vi "Export - Buffered Rx Packet.vi"(8 "error in (no error)":errorcluster, 11 "Device Item Ref in":T10 format="%.0x") -> (0 "error out":errorcluster, 3 "Rx Packet":T1 {"targetPriority" min=-2 max=16 step=1; "targetProcessor" min=-2 max=16 step=1; "Endianness" items=["big-endian"=0, "little-endian"=2]})   [LabVIEW 2019, in "UDP-Custom-Device System Explorer.lvlib"]
uses:
  UDP-Custom-Device System Explorer.lvlib
  <vilib>/NI VeriStand/Custom Device API/Custom Device Item Ref.ctl
  Types/XML - New/ImpExp - Rx Packet Data.ctl
  <vilib>/NI VeriStand/Custom Device API/Custom Device Item Info.ctl
  Shared/Types/Shared - Channel Data Type.ctl
  Shared/Types/Shared - Buffered.PacketInfo.ctl
  Shared/Types/Shared - Pointer Encoding.ctl
  Shared/Types/Shared - Receive Buffer Options.ctl
  Shared/Types/Shared - Transmit Buffer Options.ctl
  Shared/Types/Shared - New Data Options.ctl
  Shared/Types/Shared - Thread Management.ctl
  Shared/UDP-Custom-Device Shared.lvlib
  <vilib>/NI VeriStand/Custom Device API/Custom Device API.lvlib
  Property Accessors/Shared Packet Accessors.lvlib
  Property Accessors/Rx Packet Accessors.lvlib
  Property Accessors/Buffered Data Packet.lvlib
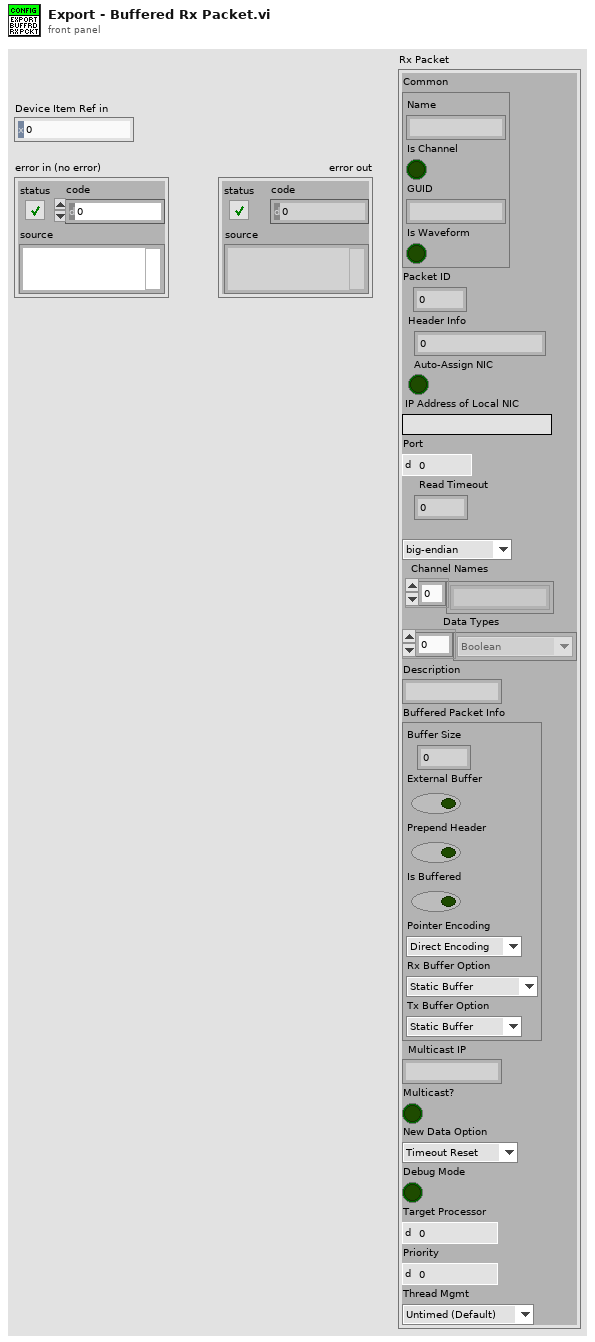
[diagram p1: front panel]
types:
  T1 = typedef "UDP-Custom-Device System Explorer.lvlib/ImpExp - Rx Packet Data.ctl" = cluster{"Common":T2, "Packet ID":i32, "Header Info":u32, "Auto-Assign NIC":bool, "IP Address of Local NIC":string, "Port":u16, "Read Timeout":i32, "Endianness":u16, "Channel Names":string[], "Data Types":T3[], "Description":string, "Buffered Packet Info":T4, "Multicast IP":string, "Multicast?":bool, "New Data Option":T8, "Debug Mode":bool, "targetProcessor":i8, "targetPriority":i16, "Thread Mgmt":T9}
  T2 = typedef "Custom Device API.lvlib/Custom Device Item Info.ctl" = cluster{"Name":string, "Is Channel":bool, "GUID":string, "Is Waveform":bool}
  T3 = typedef "UDP-Custom-Device Shared.lvlib/Shared - Channel Data Type.ctl" = enum16{"Boolean", "Single", "Double", "I8", "I16", "I32", "I64", "U8", "U16", "U32", "U64"}
  T4 = typedef "UDP-Custom-Device Shared.lvlib/Shared - Buffered.PacketInfo.ctl" = cluster{"Buffer Size":i32, "External Buffer":bool, "Prepend Header":bool, "Is Buffered":bool, "Pointer Encoding":T5, "Rx Buffer Option":T6, "Tx Buffer Option":T7}
  T5 = typedef "UDP-Custom-Device Shared.lvlib/Shared - Pointer Encoding.ctl" = enum16{"Direct Encoding", "Conversion Encoding"}
  T6 = typedef "UDP-Custom-Device Shared.lvlib/Shared - Receive Buffer Options.ctl" = enum16{"Static Buffer", "Circular Buffer", "Circular Buffer + Size", "Internal Cache", "Internal Cache + Size", "Ping Pong", "Ping Pong + Size"}
  T7 = typedef "UDP-Custom-Device Shared.lvlib/Shared - Transmit Buffer Options.ctl" = enum16{"Static Buffer", "FIFO Buffer", "FIFO Buffer + Port"}
  T8 = typedef "UDP-Custom-Device Shared.lvlib/Shared - New Data Options.ctl" = enum16{"Timeout Reset", "Counter"}
  T9 = typedef "UDP-Custom-Device Shared.lvlib/Shared - Thread Management.ctl" = enum16{"Untimed (Default)", "Timed (High Priority)"}
  T10 = typedef "Custom Device API.lvlib/Custom Device Item Ref.ctl" = u64
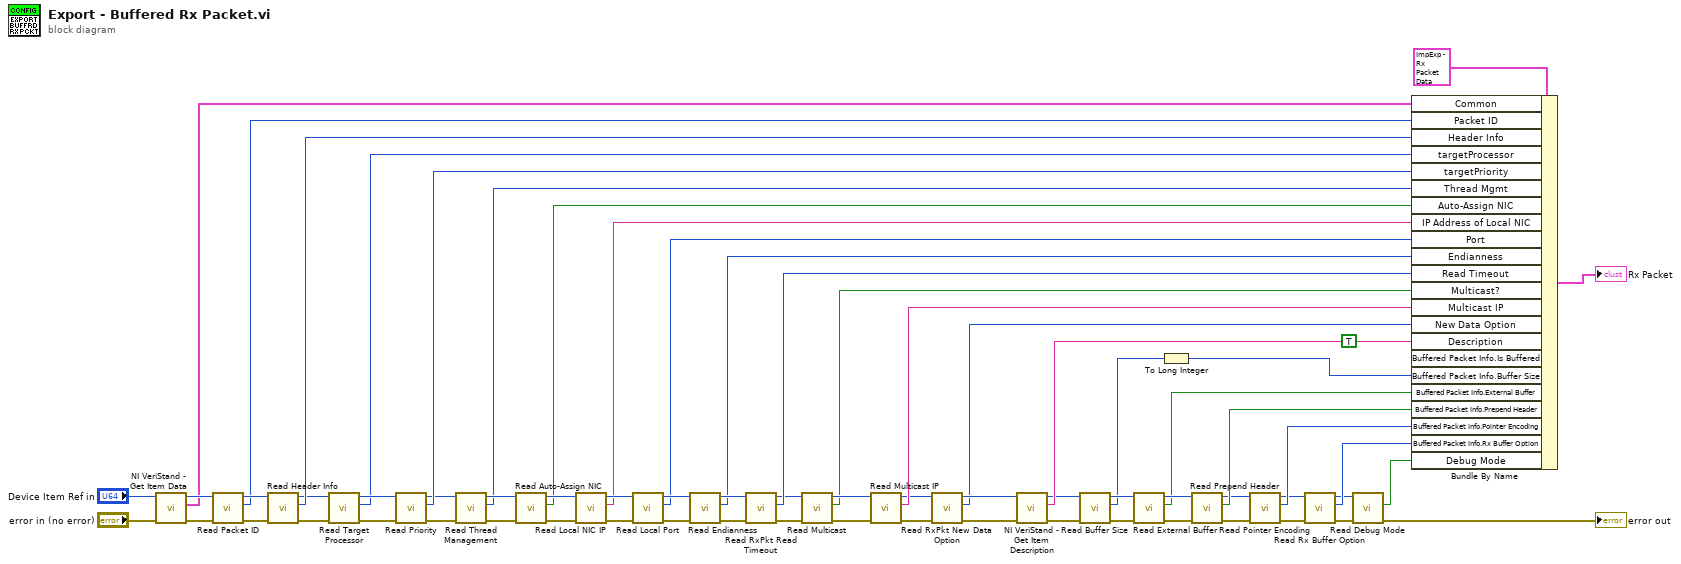
[diagram p0: block diagram]
diagram:
  n1 = call <vilib>:"NI VeriStand - Get Item Data.vi"("error in (no error)"="error in (no error)", "Item Ref in"="Device Item Ref in") -> ("error out"=w64:errorcluster, "Item Info"=w53:T2, "Item Ref out"=w57:T10)  [unwired: 6 in, 1 out]
  n2 = call "Read Packet ID.vi"("error in (no error)"=w64, "Node Ptr"=w57) -> ("error out"=w59:errorcluster, "Packet ID"=w52:i32, "Node Ptr out"=w58:T10)  [unwired: 7 in]
  n3 = call "Read Header Info.vi"("error in (no error)"=w59, "Node Ptr"=w58) -> ("error out"=w8:errorcluster, "Header Info"=w51:u32, "Node Ptr out"=w9:T10)  [unwired: 7 in]
  n4 = call "Read Target Processor.vi"("error in (no error)"=w8, "Node Ptr"=w9) -> ("error out"=w10:errorcluster, "targetProcessor"=w7:i8, "Node Ptr out"=w11:T10)  [unwired: 7 in]
  n5 = call "Read Priority.vi"("error in (no error)"=w10, "Node Ptr"=w11) -> ("error out"=w3:errorcluster, "targetPriority"=w6:i16, "Node Ptr out"=w5:T10)  [unwired: 7 in]
  n6 = call "Read Thread Management.vi"("error in (no error)"=w3, "Node Ptr"=w5) -> ("error out"=w2:errorcluster, "Thread Management"=w1:T9, "Node Ptr out"=w4:T10)  [unwired: 7 in]
  n7 = call "Read Auto-Assign NIC.vi"("error in (no error)"=w2, "Node Ptr"=w4) -> ("error out"=w63:errorcluster, "Auto-Assign NIC"=w50:bool, "Node Ptr out"=w60:T10)  [unwired: 7 in]
  n8 = call "Read Local NIC IP.vi"("error in (no error)"=w63, "Node Ptr"=w60) -> ("error out"=w62:errorcluster, "IP Address of Local NIC"=w49:string, "Node Ptr out"=w61:T10)  [unwired: 7 in]
  n9 = call "Read Local Port.vi"("error in (no error)"=w62, "Node Ptr"=w61) -> ("error out"=w65:errorcluster, "Port"=w48:u16, "Node Ptr out"=w66:T10)  [unwired: 7 in]
  n10 = call "Read Endianness.vi"("error in (no error)"=w65, "Node Ptr"=w66) -> ("error out"=w67:errorcluster, "Endianness"=w47:u16, "Node Ptr out"=w68:T10)  [unwired: 7 in]
  n11 = call "Read RxPkt Read Timeout.vi"("error in (no error)"=w67, "Node Ptr"=w68) -> ("error out"=w27:errorcluster, "Read Timeout"=w46:i32, "Node Ptr out"=w28:T10)  [unwired: 7 in]
  n12 = call "Read Multicast.vi"("error in (no error)"=w27, "Node Ptr"=w28) -> ("error out"=w31:errorcluster, "Multicast"=w30:bool, "Node Ptr out"=w32:T10)  [unwired: 7 in]
  n13 = call "Read Multicast IP.vi"("error in (no error)"=w31, "Node Ptr"=w32) -> ("error out"=w21:errorcluster, "Multicast IP Address"=w29:string, "Node Ptr out"=w23:T10)  [unwired: 7 in]
  n14 = call "Read RxPkt New Data Option.vi"("error in (no error)"=w21, "Node Ptr"=w23) -> ("error out"=w20:errorcluster, "New Data Option"=w19:T8, "Node Ptr out"=w22:T10)  [unwired: 7 in]
  n15 = call <vilib>:"NI VeriStand - Get Item Description.vi"("error in (no error)"=w20, "Item Ref in"=w22) -> ("error out"=w38:errorcluster, "Description"=w45:string, "Item Ref out"=w43:T10)  [unwired: 6 in, 1 out]
  n16 = call "Read Buffer Size.vi"("error in (no error)"=w38, "Node Ptr"=w43) -> ("error out"=w40:errorcluster, "Buffer Size"=w37:u32, "Node Ptr out"=w42:T10)  [unwired: 7 in]
  n17 = call "Read External Buffer.vi"("error in (no error)"=w40, "Node Ptr"=w42) -> ("error out"=w39:errorcluster, "External Buffer"=w36:bool, "Node Ptr out"=w41:T10)  [unwired: 7 in]
  n18 = To Long Integer(number=w37) -> (32bit integer=w33:i32)
  n19 = call "Read Prepend Header.vi"("error in (no error)"=w39, "Node Ptr"=w41) -> ("error out"=w25:errorcluster, "Prepend Header"=w35:bool, "Node Ptr out"=w26:T10)  [unwired: 7 in]
  n20 = call "Read Pointer Encoding.vi"("error in (no error)"=w25, "Node Ptr"=w26) -> ("error out"=w17:errorcluster, "Pointer Encoding"=w24:T5, "Node Ptr out"=w18:T10)  [unwired: 7 in]
  n21 = call "Read Rx Buffer Option.vi"("error in (no error)"=w17, "Node Ptr"=w18) -> ("error out"=w14:errorcluster, "Buffer Option"=w16:T6, "Node Ptr out"=w15:T10)  [unwired: 7 in]
  n22 = call "Read Debug Mode.vi"("error in (no error)"=w14, "Node Ptr"=w15) -> ("error out"=→"error out":errorcluster, "Debug Mode"=w12:bool)  [unwired: 7 in, 1 out]
  n23 = Bundle By Name(cluster=T1 {"Common"={"Name"="", "Is Channel"=FALSE, "GUID"="", "Is Waveform"=FALSE}, "Packet ID"=0, "Header Info"=0, "Auto-Assign NIC"=FALSE, "IP Address of Local NIC"="", "Port"=0, "Read Timeout"=0, "Endianness"=0, "Channel Names"=[], "Data Types"=[], "Description"="", "Buffered Packet Info"={"Buffer Size"=0, "External Buffer"=FALSE, "Prepend Header"=FALSE, "Is Buffered"=FALSE, "Pointer Encoding"=enum."Direct Encoding", "Rx Buffer Option"=enum."Static Buffer", "Tx Buffer Option"=enum."Static Buffer"}, "Multicast IP"="", "Multicast?"=FALSE, "New Data Option"=enum."Timeout Reset", "Debug Mode"=FALSE, "targetProcessor"=0, "targetPriority"=0, "Thread Mgmt"=enum."Untimed (Default)"} ("Rx Packet"), "Common"=w53, "Packet ID"=w52, "Header Info"=w51, "targetProcessor"=w7, "targetPriority"=w6, "Thread Mgmt"=w1, "Auto-Assign NIC"=w50, "IP Address of Local NIC"=w49, "Port"=w48, "Endianness"=w47, "Read Timeout"=w46, "Multicast?"=w30, "Multicast IP"=w29, "New Data Option"=w19, "Description"=w45, "Buffered Packet Info.Is Buffered"=TRUE, "Buffered Packet Info.Buffer Size"=w33, "Buffered Packet Info.External Buffer"=w36, "Buffered Packet Info.Prepend Header"=w35, "Buffered Packet Info.Pointer Encoding"=w24, "Buffered Packet Info.Rx Buffer Option"=w16, "Debug Mode"=w12) -> (→"Rx Packet":T1)
